vi "Rx FIFOs.vi"(0 "rx.fifo":refnum<k21>, 1 "rx.data sink":enum16{"SFP Port 0", "SFP Port 1", "Host"}(ring)=enum."SFP Port 1", 5 "rx.host fifo":refnum<k21>, 7 "rx.sfp fifo":refnum<k21>) -> ()   [LabVIEW 2016]
uses:
  <vilib>/rvi/DataTransferAndStorage/Container/Common/niFpgaContainerExecOnDevCompGetState.vi
  <vilib>/rvi/Emulation/niFpgaEmulationIsFPGAContextNoSignature.vi
  <vilib>/rvi/Emulation/niFpgaSctlEmulationGetInTimedLoop.vi
  <vilib>/rvi/errors/niFpgaSetErrorForExecOnDevCompSimple.vi
  <vilib>/rvi/eio/common/nirviEmuReportErrorAndStop.vi
  <vilib>/rvi/DataTransferAndStorage/Container/Common/niFpgaContainerGetUniqueNameForEmu.vi
  <vilib>/rvi/FIFO/Fifo_Resource/nirvififoEmulationSetSize.vi
  <vilib>/rvi/FIFO/Fifo_Resource/nirviFifoEmulationQueueMgr.vi
  <instcachedir>/0/nirviFifoEmulationQueueMgr_E5CAEC123FF24DC58D834DCA3CDAA9B5.lvgen/nirviFifoEmulationQueueMgr_E5CAEC123FF24DC58D834DCA3CDAA9B5_004.vi
  <vilib>/rvi/FIFO/Fifo_Resource/nirvififoEmulationDetermineInputValidOut.vi
  <vilib>/rvi/FIFO/Fifo_Resource/nirvififoEmulationCreateLock.vi
  <vilib>/rvi/Emulation/niFpgaProcessEmulError.vi
  <vilib>/rvi/FIFO/Fifo_Resource/nirvififoEmulationObtainLock.vi
  <vilib>/rvi/FIFO/Fifo_Resource/nirvififoEmulationReleaseLock.vi
  <vilib>/rvi/occurrence/nirviWaitOnOccurrenceBase.vi
  <vilib>/rvi/errors/nirviReportUnexpectedCaseInternalError.vi
  <vilib>/rvi/errors/nirviReportUnexpectedCaseInternalError (U32).vi
  <vilib>/Utility/error.llb/Clear Errors.vi
  <vilib>/rvi/interface/RandomDataEmulation/niFpgaRandomDataHandleErrors.vi
  <instcachedir>/0/nirviFifoEmulationQueueMgr_E5CAEC123FF24DC58D834DCA3CDAA9B5.lvgen/nirviFifoEmulationQueueMgr_E5CAEC123FF24DC58D834DCA3CDAA9B5_003.vi
  <vilib>/rvi/DataTransferAndStorage/Container/XNode/niFpgaContainer.xnode
  <vilib>/rvi/FIFO/Fifo_Resource/niFpgaFifoEmulationRefIn.vi
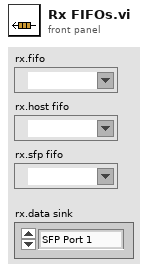
[diagram p1: front panel]
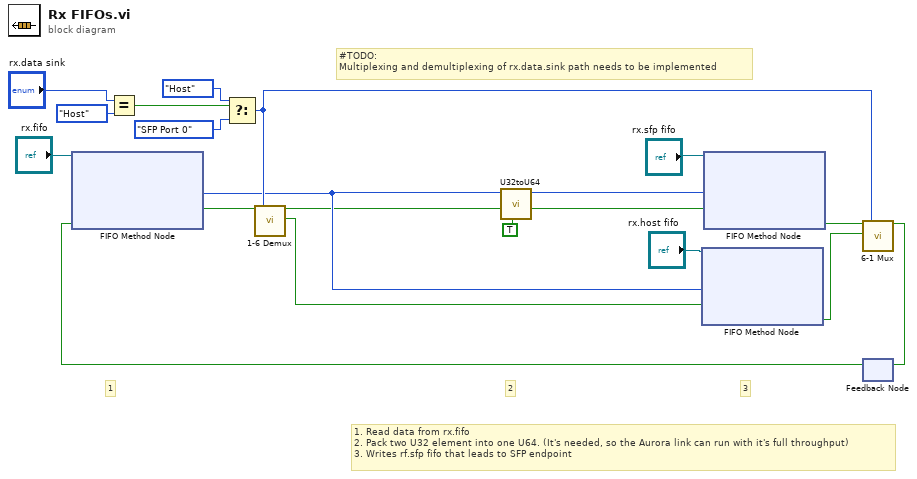
[diagram p0: block diagram]
diagram:
  # "3"
  # "2"
  # "1"
  # "1. Read data from rx.fifo\n2. Pack two U32 element into one U64. (It's needed, so the Aurora link can run with it's full throughput)\n3. Writes rf.sfp fifo that leads to SFP endpoint"
  # "#TODO:\nMultiplexing and demultiplexing of rx.data.sink path needs to be implemented"
  n1 = Equal?(x="rx.data sink", y=enum16{"SFP Port 0", "SFP Port 1", "Host"}."Host") -> (x = y?=w11:bool)
  n2 = Select(t=enum16{"SFP Port 0", "SFP Port 1", "Host"}."Host" ("y"), s=w11, f=enum16{"SFP Port 0", "SFP Port 1", "Host"}."SFP Port 0" ("y")) -> (s? t:f=w7:enum16{"SFP Port 0", "SFP Port 1", "Host"})
  n3 = feedback #1() -> (w19:bool)  [unwired: 1 in]
  n4 = xnode ("FIFO Method Node")("Ready for Output"=w19, "FIFO In"="rx.fifo") -> ("Element"=w5:u32, "Output Valid"=w14:bool)  [unwired: 1 out]
  n5 = call "1-6 Demux.vi"("input"=w14, "select"=w7) -> ("output 0"=w2:bool, "output 2"=w6:bool)  [unwired: 12 in, 4 out]
  n6 = call "U32toU64.vi"("ready for output"=TRUE, "input valid"=w2, "U32 in"=w5) -> ("output valid"=w3:bool, "U64 out"=w4:u64)  [unwired: 6 in, 1 out]
  n7 = xnode ("FIFO Method Node")("Element"=w5, "Input Valid"=w6, "FIFO In"="rx.host fifo") -> ("Ready for Input"=w13:bool)  [unwired: 1 out]
  n8 = xnode ("FIFO Method Node")("Element"=w4, "Input Valid"=w3, "FIFO In"="rx.sfp fifo") -> ("Ready for Input"=w15:bool)  [unwired: 1 out]
  n9 = call "6-1 Mux.vi"("input 0"=w15, "input 2"=w13, "select"=w7) -> ("output"=w20:bool)  [unwired: 16 in]
  n10 = feedback-in #1(w20) -> ()
